vi "GetExcelAllData.vi"(8 "error in":errorcluster, 11 "template (empty)":path) -> (0 "error out":errorcluster, 2 "data":string[][](array[string]))   [LabVIEW 2016]
uses:
  <vilib>/addons/_office/excel.llb/Excel Get Data ([str]).vi
  <vilib>/Utility/NIReport.llb/NI_report.lvclass
  <vilib>/addons/_office/NI_ReportGenerationToolkit.lvlib
  <vilib>/Utility/NIReport.llb/Excel/NI_Excel.lvclass
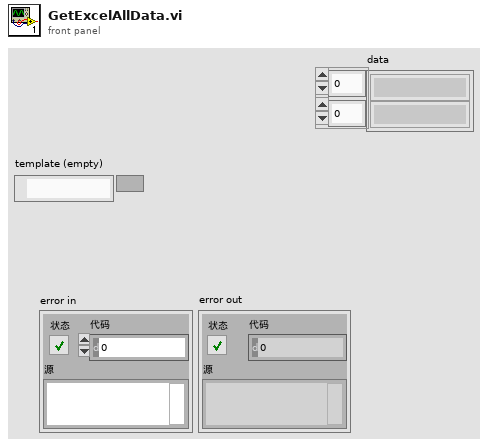
[diagram p1: front panel]
types:
  T1 = enum16{"Standard Report", "HTML", "Word", "Excel"}
  T2 = enum16{"maximized", "minimized", "normal", "no change"}
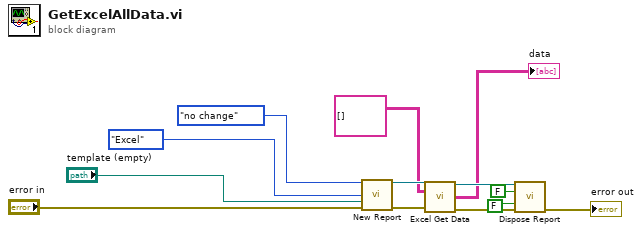
[diagram p0: block diagram]
diagram:
  n1 = call <vilib>:"New Report.vi"("window state (normal)"=T2."no change", "report type"=T1."Excel", "template (empty)"="template (empty)", "error in (no error)"="error in") -> ("report out"=w9:refnum<class "NI_report.lvclass">, "error out"=w10:errorcluster)  [unwired: 10 in]
  n2 = call-poly <vilib>:"Excel Get Data.vi"("report in"=w9, "data type"=string[][] [], "error in (no error)"=w10) -> ("report out"=w7:refnum<class "NI_report.lvclass">, "data"=→"data":string[][], "error out"=w8:errorcluster)  [unwired: 10 in]
  n3 = call-dynamic "Dispose Report.vi"("report in"=w7, "wait until printing completed? (T)"=FALSE, "save changes? (F)"=FALSE, "error in (no error)"=w8) -> ("error out"=→"error out":errorcluster)  [unwired: 11 in]
